vi "AddFuction_EnDisable.vi"(8 "error in (no error)":errorcluster, 11 "Value":T1) -> (3 "Selected Param":variant)   [LabVIEW 2019]
uses:
  Controls/UI_Process_Type.ctl
  Controls/Control_EnDisable_Action.ctl
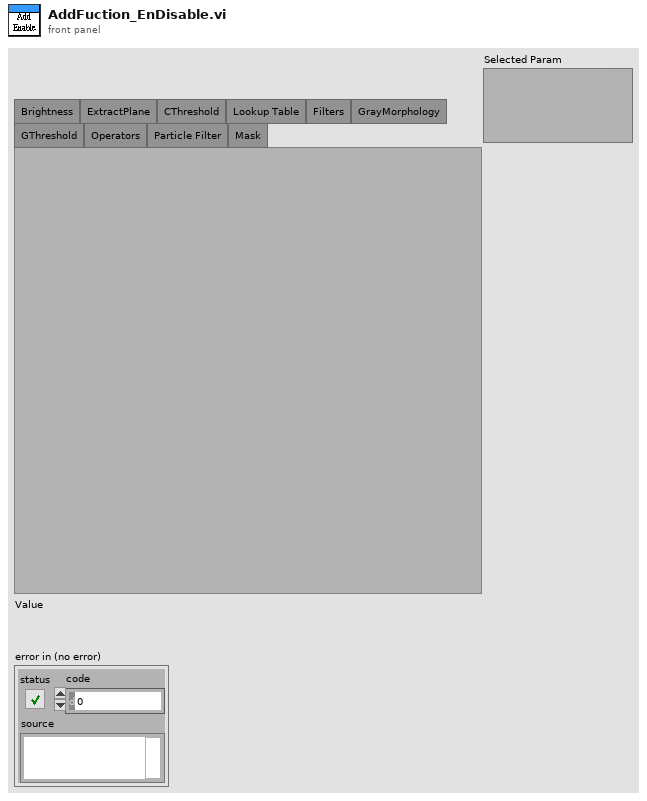
[diagram p1: front panel]
types:
  T1 = typedef "UI_Process_Type.ctl" = enum32{"None", "Brightness", "ExtractPlane", "CThreshold", "Lookup Table", "Filters", "GrayMorphology", "GThreshold", "Operators", "Particle Filter", "Mask"}
  T2 = typedef "Control_EnDisable_Action.ctl" = enum16{"Store Ref", "Add Mode", "Select Mode", "Enable All", "OnePageEnable", "OnePageDisable", "AllPageDisable", "AllPageEnable", "PageRefOut"}
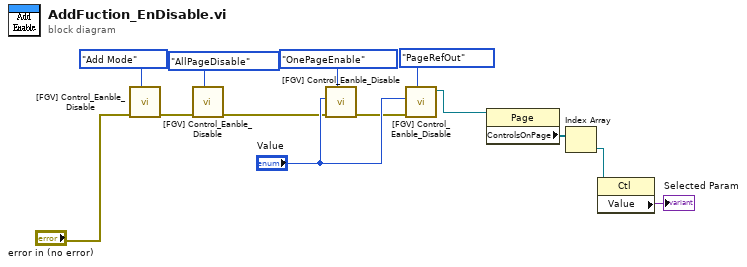
[diagram p0: block diagram]
diagram:
  n1 = call "[FGV] Control_Eanble_Disable.vi"("Control_EnDisable_Action"=Control_EnDisable_Action."Add Mode", "Error In"="error in (no error)") -> ("Error Out"=w7:errorcluster)  [unwired: 8 in, 1 out]
  n2 = call "[FGV] Control_Eanble_Disable.vi"("Control_EnDisable_Action"=Control_EnDisable_Action."AllPageDisable", "Error In"=w7) -> ("Error Out"=w9:errorcluster)  [unwired: 8 in, 1 out]
  n3 = call "[FGV] Control_Eanble_Disable.vi"("Control_EnDisable_Action"=Control_EnDisable_Action."OnePageEnable", "Error In"=w9, "Tab"="Value") -> ("Error Out"=w11:errorcluster)  [unwired: 7 in, 1 out]
  n4 = call "[FGV] Control_Eanble_Disable.vi"("Control_EnDisable_Action"=Control_EnDisable_Action."PageRefOut", "Error In"=w11, "Tab"="Value") -> ("PageRefOut"=w2:refnum<vi>)  [unwired: 7 in, 1 out]
  n5 = property class="Page"(reference=w2) -> ("ControlsOnPage"=w4:refnum<vi>[])  [unwired: 1 in, 2 out]
  n6 = Index Array(array=w4) -> (element=w3:refnum<vi>)  [unwired: 1 in]
  n7 = property class="Ctl"(reference=w3) -> ("Value"=→"Selected Param":variant)  [unwired: 1 in, 2 out]
